vi "Pass Through Device State Information.vi"(8 "error in":errorcluster, 10 "Device State Information":T1, 11 "EMS in":refnum<class "EMS.lvclass">) -> (0 "error out":errorcluster, 3 "EMS out":refnum<class "EMS.lvclass">)   [LabVIEW 2018, in "EMS Core.lvlib" / "EMS.lvclass"]
uses:
  EMS.lvclass
  C:/Program Files (x86)/National Instruments/LabVIEW 2018/vi.lib/ActorFramework/Actor/Actor.lvclass
  C:/Users/Administrator/Desktop/LabVIEW EMS/EMS Generic Actor/EMS Generic/EMS Generic.lvclass
  EMS Generic Actor/EMS Generic/Controls/Device Information Cluster.ctl
  EMS Generic Actor/EMS Generic/Controls/Device State.ctl
  <vilib>/ActorFramework/Actor/Actor.lvclass/Actor.ctl
  EMS Generic Actor/EMS Generic/EMS Generic.lvclass/EMS Generic.ctl
  EMS Generic Actor/EMS Generic Messages/Device State Information Msg/Device State Information Msg.lvclass/Device State Information Msg.ctl
  <vilib>/ActorFramework/Message Enqueuer/Message Enqueuer.lvclass/Message Enqueuer.ctl
  <vilib>/ActorFramework/Message Enqueuer/Enqueue.vi
  EMS Generic Actor/EMS Generic Messages/Device State Information Msg/Device State Information Msg.lvclass
  C:/Program Files (x86)/National Instruments/LabVIEW 2018/vi.lib/ActorFramework/Message/Message.lvclass
  <vilib>/ActorFramework/Message Priority Queue/Priority Enqueue.vi
  EMS Generic Actor/EMS Generic/EMS Generic.lvclass
  <vilib>/ActorFramework/Actor/Actor.lvclass
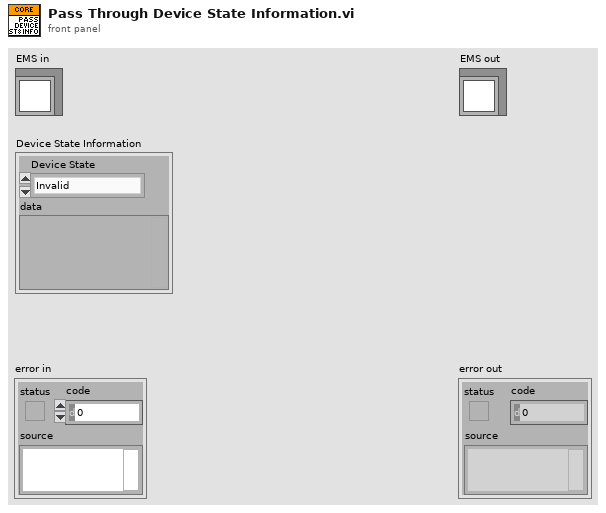
[diagram p1: front panel]
types:
  T1 = typedef "EMS Generic Actor.lvlib/EMS Generic.lvclass/Device Information Cluster.ctl" = cluster{"Device State":T2, "data":variant}
  T2 = typedef "EMS Generic Actor.lvlib/EMS Generic.lvclass/Device State.ctl" = enum16{"Invalid", "Clear", "DevIDs in Config", "DevIDs on uGrid", "DevIDs not on uGrid", "Update IED_Status", "Update DER_Status", "Update DER_Measurement", "Update SmartRelay_Measurement"}
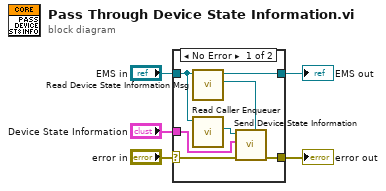
[diagram p0: block diagram]
diagram:
  n1 = case shown="No Error" "error in" {
    selector: "error in" -> [w7 w14]
    tunnel: [w6 w14] -> w4
    tunnel: [w10 w13] -> w2
    tunnel: "EMS in" -> [w11 w13]
    tunnel: "Device State Information" -> [w8 _]
    frame No Error {
      n2 = call "Read Device State Information Msg.vi"("EMS Generic"=w11) -> ("Return Device State Information Msg"=w12:refnum<class "Device State Information Msg.lvclass">, "dup EMS Generic"=w10:refnum<class "EMS.lvclass">)  [unwired: 9 in]
      n3 = call <vilib>:"Read Caller Enqueuer.vi"("Actor"=w11) -> ("Caller Enqueuer"=w9:refnum<class "Message Enqueuer.lvclass">)  [unwired: 10 in]
      n4 = call "Send Device State Information.vi"("Message Type"=w12, "error in (no error)"=w7, "Action Engine"=w8, "Message Enqueuer"=w9) -> ("error out"=w6:errorcluster)  [unwired: 6 in, 1 out]
    }
    frame Error {
    }
  }
  "error out" <- w4
  "EMS out" <- w2
